vi "checkForHPTimeouts.vi"(8 "error in (no error)":errorcluster, 11 "ILCCommunications in":refnum<class "ILCCommunications.lvclass">) -> (0 "error out":errorcluster, 2 "IDs":i32[](array[numeric]), 3 "ILCCommunications out":refnum<class "ILCCommunications.lvclass">)   [LabVIEW 2016, in "ILCCommunications.lvclass"]
uses:
  ILCCommunications.lvclass
  ILCCommunications.lvclass/ILCCommunications.ctl
  Common_RT_Modbus/DataTypes/ExceptionCodes.ctl
  Common_RT_HPILC/HPILC/HPILC.lvclass/HPILC.ctl
  Common_RT_ILC/ILC/ILC.lvclass/ILC.ctl
  Common_RT_HPILC/HPILC/HPILC.lvclass
  D:/Code/ts_M1M3Support/Common_RT_ILC/ILC/ILC.lvclass
  Common_RT_Modbus/RTModbus.lvlib
  Common_RT_ILC/ILC/ILC.lvclass
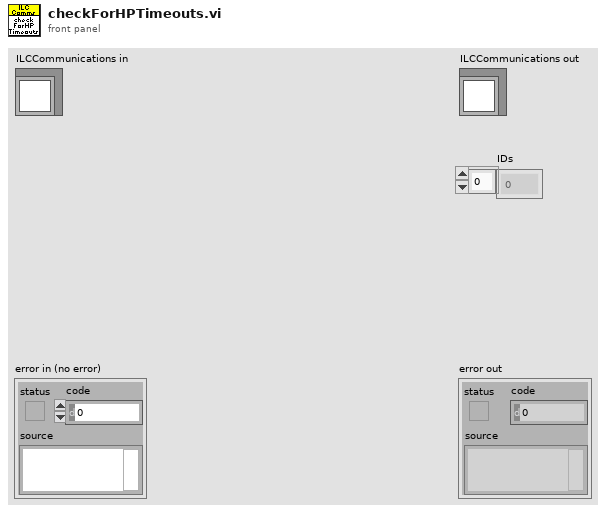
[diagram p1: front panel]
types:
  T1 = typedef "RTModbus.lvlib/ExceptionCodes.ctl" = u16
  T2 = typedef "RTILC.lvlib/ILCData.ctl" = cluster{"Constants":T3, "Command":T4, "Telemetry":T6, "Responses":T7, "Timestamps":T8, "Timings":T9}
  T3 = typedef "RTILC.lvlib/ILCConstants.ctl" = cluster{"Subnet":u8, "Address":u8}
  T4 = typedef "RTILC.lvlib/ILCCommand.ctl" = cluster{"Mode":u16, "TemporaryAddress":u8, "ADCScanRate":T5, "ADCChannel":u8, "ADCOffset":sgl, "ADCSensitivity":sgl}
  T5 = typedef "RTILC.lvlib/ILCScanRates.ctl" = u8
  T6 = typedef "RTILC.lvlib/ILCTelemetry.ctl" = cluster{"UniqueID":u64, "FirmwareType":u8, "NetworkNodeType":u8, "ILCOption":u8, "NetworkNodeOption":u8, "MajorRevision":u8, "MinorRevision":u8, "FirmwareName":string, "Mode":u16, "MajorFault":bool, "MinorFault":bool, "FaultOverride":bool, "MainCalibrationError":bool, "BackupCalibrationError":bool, "UniqueIDCRCMismatch":bool, "AppTypeNodeTypeMismatch":bool, "AppMissing":bool, "AppCRCMismatch":bool, "TEDSNotFound":bool, "TEDS1Mismatch":bool, "TEDS2Mismatch":bool, "WatchdogResetDetected":bool, "BrownoutDetected":bool, "EventTrapResetDetected":bool, "MotorPowerFault":bool, "SSRPowerFault":bool, "AuxPowerFault":bool, "SMCPowerFault":bool, "TemporaryAddress":u8, "ADCScanRate":T5, "MainADCCalibrationK":sgl[], "MainSensorOffset":sgl[], "MainSensorSensitivity":sgl[], "BackupADCCalibrationK":sgl[], "BackupSensorOffset":sgl[], "BackupSensorSensitivity":sgl[]}
  T7 = typedef "RTILC.lvlib/ILCResponses.ctl" = cluster{"ReportServerID":T1, "ReportServerStatus":T1, "Mode":T1, "TemporaryAddress":T1, "Reset":T1, "ADCScanRate":T1, "ADCOffsetSensitivity":T1, "ReportCalibrationData":T1}
  T8 = typedef "RTILC.lvlib/ILCTimestamps.ctl" = cluster{"ReportServerID":dbl, "ReportServerStatus":dbl, "Mode":dbl, "TemporaryAddress":dbl, "Reset":dbl, "ADCScanRate":dbl, "ADCOffsetSensitivity":dbl, "ReportCalibrationData":dbl}
  T9 = typedef "RTILC.lvlib/ILCTimings.ctl" = cluster{"ReportServerID":u32, "ReportServerStatus":u32, "Mode":u32, "TemporaryAddress":u32, "Reset":u32, "ADCScanRate":u32, "ADCOffsetSensitivity":u32, "ReportCalibrationData":u32}
  T10 = typedef "RTHPILC.lvlib/HPData.ctl" = cluster{"Constants":T11, "Command":T12, "Telemetry":T13, "Responses":T14, "Timings":T15, "Timestamps":T16}
  T11 = typedef "RTHPILC.lvlib/HPConstants.ctl" = cluster{"ID":i16, "ReferencePosition":i32, "XPosition":sgl, "YPosition":sgl, "ZPosition":sgl}
  T12 = typedef "RTHPILC.lvlib/HPCommand.ctl" = cluster{"Steps":i8}
  T13 = typedef "RTHPILC.lvlib/HPTelemetry.ctl" = cluster{"ILCFault":bool, "LimitSwitchCWOperated":bool, "LimitSwitchCCWOperated":bool, "BroadcastCounter":u8, "SSIEncoderValue":i32, "LoadCellForce":sgl}
  T14 = typedef "RTHPILC.lvlib/HPResponses.ctl" = cluster{"StepMotor":T1, "ForceAndStatus":T1}
  T15 = typedef "RTHPILC.lvlib/HPTimings.ctl" = cluster{"BroadcastStepMotor":u32, "ForceAndStatus":u32, "FreezeSensorValues":u32, "StepMotor":u32}
  T16 = typedef "RTHPILC.lvlib/HPTimestamps.ctl" = cluster{"StepMotor":dbl, "ForceAndStatus":dbl}
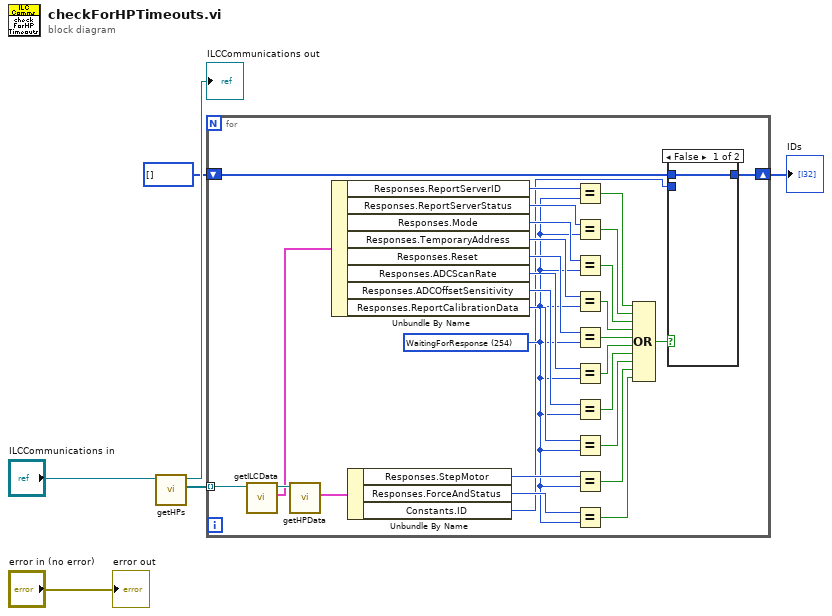
[diagram p0: block diagram]
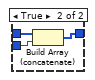
[diagram p2: hidden frame]
diagram:
  n1 = call "getHPs.vi"("ILCCommunications in"="ILCCommunications in") -> ("HPs"=w3:refnum<class "HPILC.lvclass">[], "ILCCommunications out"=→"ILCCommunications out":refnum<class "ILCCommunications.lvclass">)  [unwired: 9 in]
  n2 = for {
    tunnel: w3 -> [w35] mode=indexing
    shift-right: [w7] -> w2
    shift-left: i32[] [] ("IDs") -> [w9]
    w21 = T1 254 items=["OK"=0, "IllegalFunction"=1, "IllegalDataAddress"=2, "IllegalDataValue"=3, "SlaveDeviceFailure"=4, "Acknowledge"=5, "SlaveDeviceBusy"=6, "NegativeAcknowledge"=7, "MemoryParityError"=8, "GatewayPathUnavailable"=9, "GatewayTargetDeviceFailedToRespond"=10, "WaitingForResponse"=254, "CRCError"=255] ("y")
    n3 = call "getILCData.vi"("ILC in"=w35) -> ("ILCData"=w33:T2, "ILC out"=w34:refnum<class "HPILC.lvclass">)  [unwired: 9 in]
    n4 = call "getHPData.vi"("HPILC in"=w34) -> ("HPData"=w32:T10)  [unwired: 9 in, 1 out]
    n5 = Unbundle By Name(w33) -> ("Responses.ReportServerID"=w31:T1, "Responses.ReportServerStatus"=w30:T1, "Responses.Mode"=w29:T1, "Responses.TemporaryAddress"=w22:T1, "Responses.Reset"=w28:T1, "Responses.ADCScanRate"=w27:T1, "Responses.ADCOffsetSensitivity"=w26:T1, "Responses.ReportCalibrationData"=w25:T1)
    n6 = Unbundle By Name(w32) -> ("Responses.StepMotor"=w24:T1, "Responses.ForceAndStatus"=w23:T1, "Constants.ID"=w8:i16)
    n7 = Equal?(x=w31, y=w21) -> (x = y?=w20:bool)
    n8 = Equal?(x=w30, y=w21) -> (x = y?=w19:bool)
    n9 = Equal?(x=w29, y=w21) -> (x = y?=w18:bool)
    n10 = Equal?(x=w22, y=w21) -> (x = y?=w17:bool)
    n11 = Equal?(x=w28, y=w21) -> (x = y?=w16:bool)
    n12 = Equal?(x=w27, y=w21) -> (x = y?=w15:bool)
    n13 = Equal?(x=w26, y=w21) -> (x = y?=w14:bool)
    n14 = Equal?(x=w25, y=w21) -> (x = y?=w13:bool)
    n15 = Equal?(x=w24, y=w21) -> (x = y?=w12:bool)
    n16 = Equal?(x=w23, y=w21) -> (x = y?=w11:bool)
    n17 = Compound Arithmetic op=OR(w20, w19, w18, w17, w16, w15, w14, w13, w12, w11) -> (w10:bool)
    n18 = case shown="False" w10 {
      tunnel: w9 -> [w36 w39]
      tunnel: w8 -> [_ w38]
      tunnel: [w36 w37] -> w7
      frame False {
      }
      frame True {
        n19 = Build Array (concatenate)(w39, w38) -> (w37:i32[])
      }
    }
  }
  "IDs" <- w2
  "error out" <- "error in (no error)"
